vi "Get Path Transformation Key Names.vi"() -> (1 "VI Checksums":string="file_checksums", 2 "New Paths Key":string="file_paths.new", 3 "Original Paths Key":string="file_paths.original")   [LabVIEW 2020, in "AB_Build.lvclass"]
uses:
  <vilib>/AppBuilder/AB_Classes/Build/AB_Build.lvclass
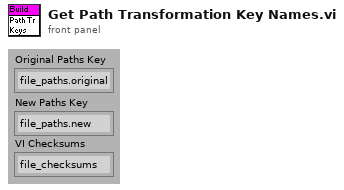
[diagram p1: front panel]
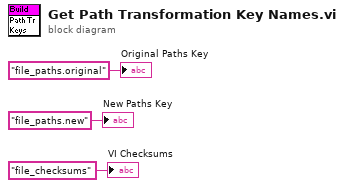
[diagram p0: block diagram]
diagram:
  "Original Paths Key" <- "file_paths.original"
  "New Paths Key" <- "file_paths.new"
  "VI Checksums" <- "file_checksums"
